vi "displayVolume.vi"(0 "frames":u16[][][](array[numeric]), 3 "z":dbl[](array[numeric]), 5 "overlay (z:-1 all planes)":cluster{"X":i32, "Y":i32, "Z":i32}[][](array[cluster]), 7 "stop immediately":bool) -> (13 "z profile":dbl[](array[numeric]), 14 "X0out":i32, 15 "deltaXout":i32, 16 "Y0out":i32, 17 "deltaYout":i32, 18 "zout (plane index)":i32 min=0 max=0)   [LabVIEW 2017]
uses:
  globalUtilities.vi
  <vilib>/Utility/file.llb/Write Delimited Spreadsheet (I64).vi
  <vilib>/Utility/file.llb/Write Delimited Spreadsheet (DBL).vi
  <vilib>/Analysis/NI_AALBase.lvlib
panel:
  in  "save marginal":bool
  in  "cut init frames":i32
  in  "refresh time (ms)":i32=200
  in  "zprof_variance":bool
  in  "save z profile":bool
  out "marginal plot":dbl[](graph)
  in  "marginal":u16(ring)=2 items=["x", "y", "none"]
  in  "z min":u16=100
  in  "z max":u16=65535
  in  "overlay depth":i32=3
  in  "overlay dotsize":i32=3
  in  "adjust y scale (to area)":bool
  out "Delta z":dbl
  in  "adjust y scale (to cursors)":bool
  out "single frame":T1(plugin-control)
  out "z profile of area":cluster{"X":dbl, "Y":dbl}[](graph)
  in  "deltaY":i32=4
  in  "deltaX":i32=8
  in  "Y0":i32=544
  in  "X0":i32=216
  out "single frame":u16[][](graph)
  in  "plane index":i32 min=0 max=37 format="%04.0f"
  out "axis-summed frame":u64[][](graph)
  in  "axis":u16(ring)=2 items=["x", "y", "z"]
  in  "stop":bool
  # "USE THIS VI TO DISPLAY A VOLUME"
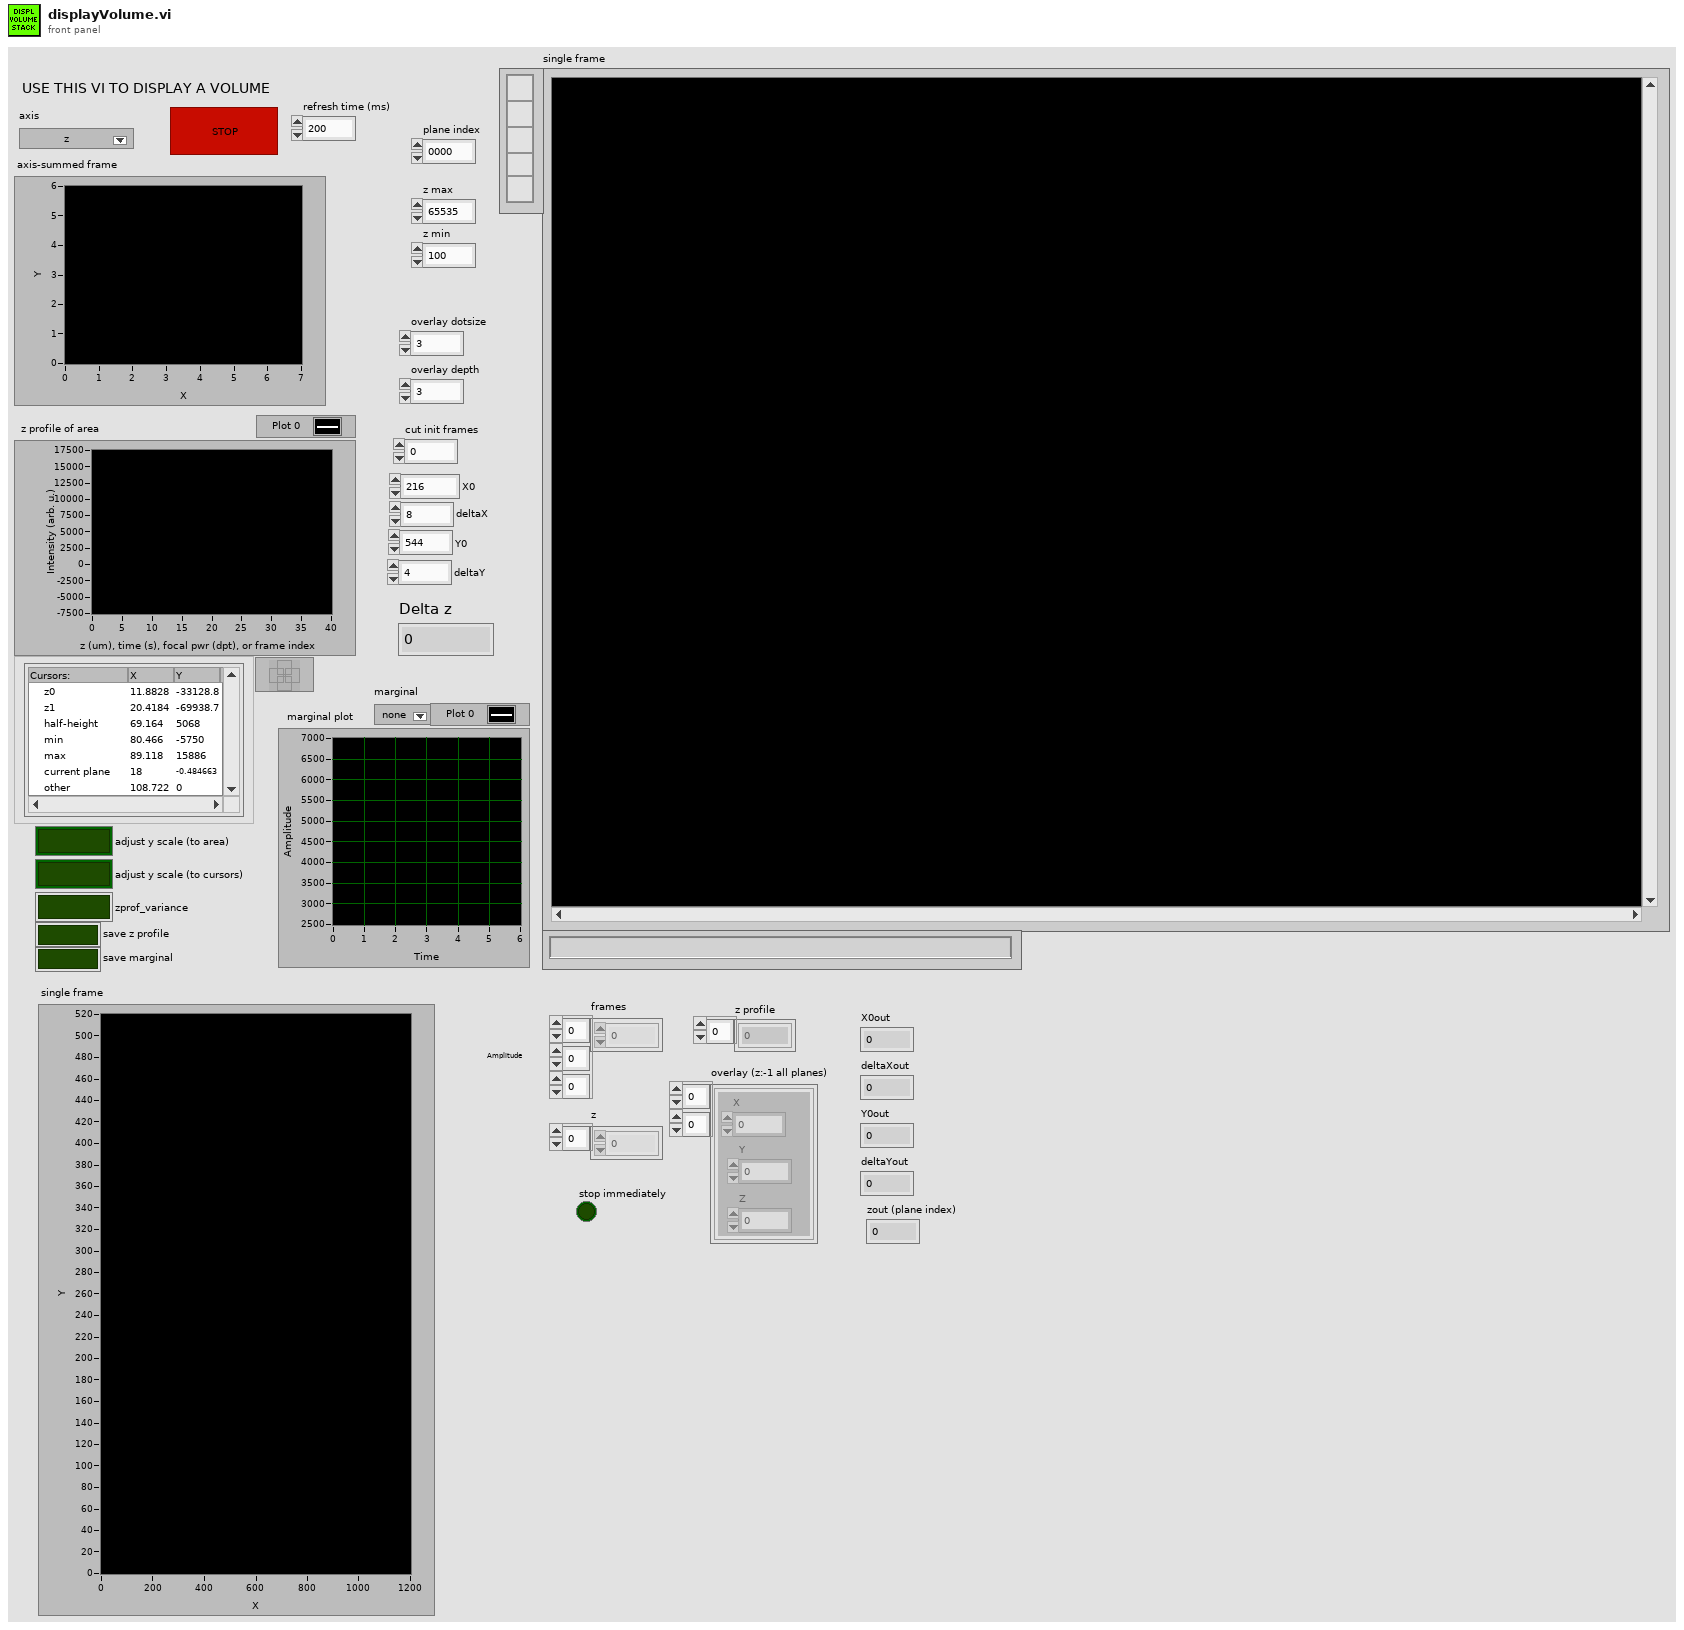
[diagram p1: front panel]
types:
  T1 = typedef "IMAQ Image.ctl" = refnum<image>
  T2 = typedef "Image Type" = u32
  T3 = typedef "LVCursorListTypeDef.ctl" = cluster{"Name":string, "Color":u32, "Style":u8, "Point Style":u8, "Name Visible":bool, "Allow Drag":bool, "Cursor Mode":u32, "Plot":i32, "Index":i32, "Position":cluster{"X":dbl, "Y":dbl}, "X Scale":u32, "Y Scale":u32, "Watch Plots":i32[], "Watch All Plots":bool, "Plot Area":i32, "Label Offset":cluster{"X":dbl, "Y":dbl}}[]
  T4 = cluster{"Name":string, "Color":u32, "Style":u8, "Point Style":u8, "Name Visible":bool, "Allow Drag":bool, "Cursor Mode":u32, "Plot":i32, "Index":i32, "Position":cluster{"X":dbl, "Y":dbl}, "X Scale":u32, "Y Scale":u32, "Watch Plots":i32[], "Watch All Plots":bool, "Plot Area":i32, "Label Offset":cluster{"X":dbl, "Y":dbl}}
  T5 = cluster{"Global Rectangle":i32[], "Contours":cluster{"Contour Type":u32, "ROI Type":u32, "Points":i32[]}[]}
  T6 = typedef "IMAQ Point" = cluster{"X":sgl, "Y":sgl}
  T7 = typedef "IMAQ Rectangle" = cluster{"Left":i32, "Top":i32, "Right":i32, "Bottom":i32, "Rotation":dbl}
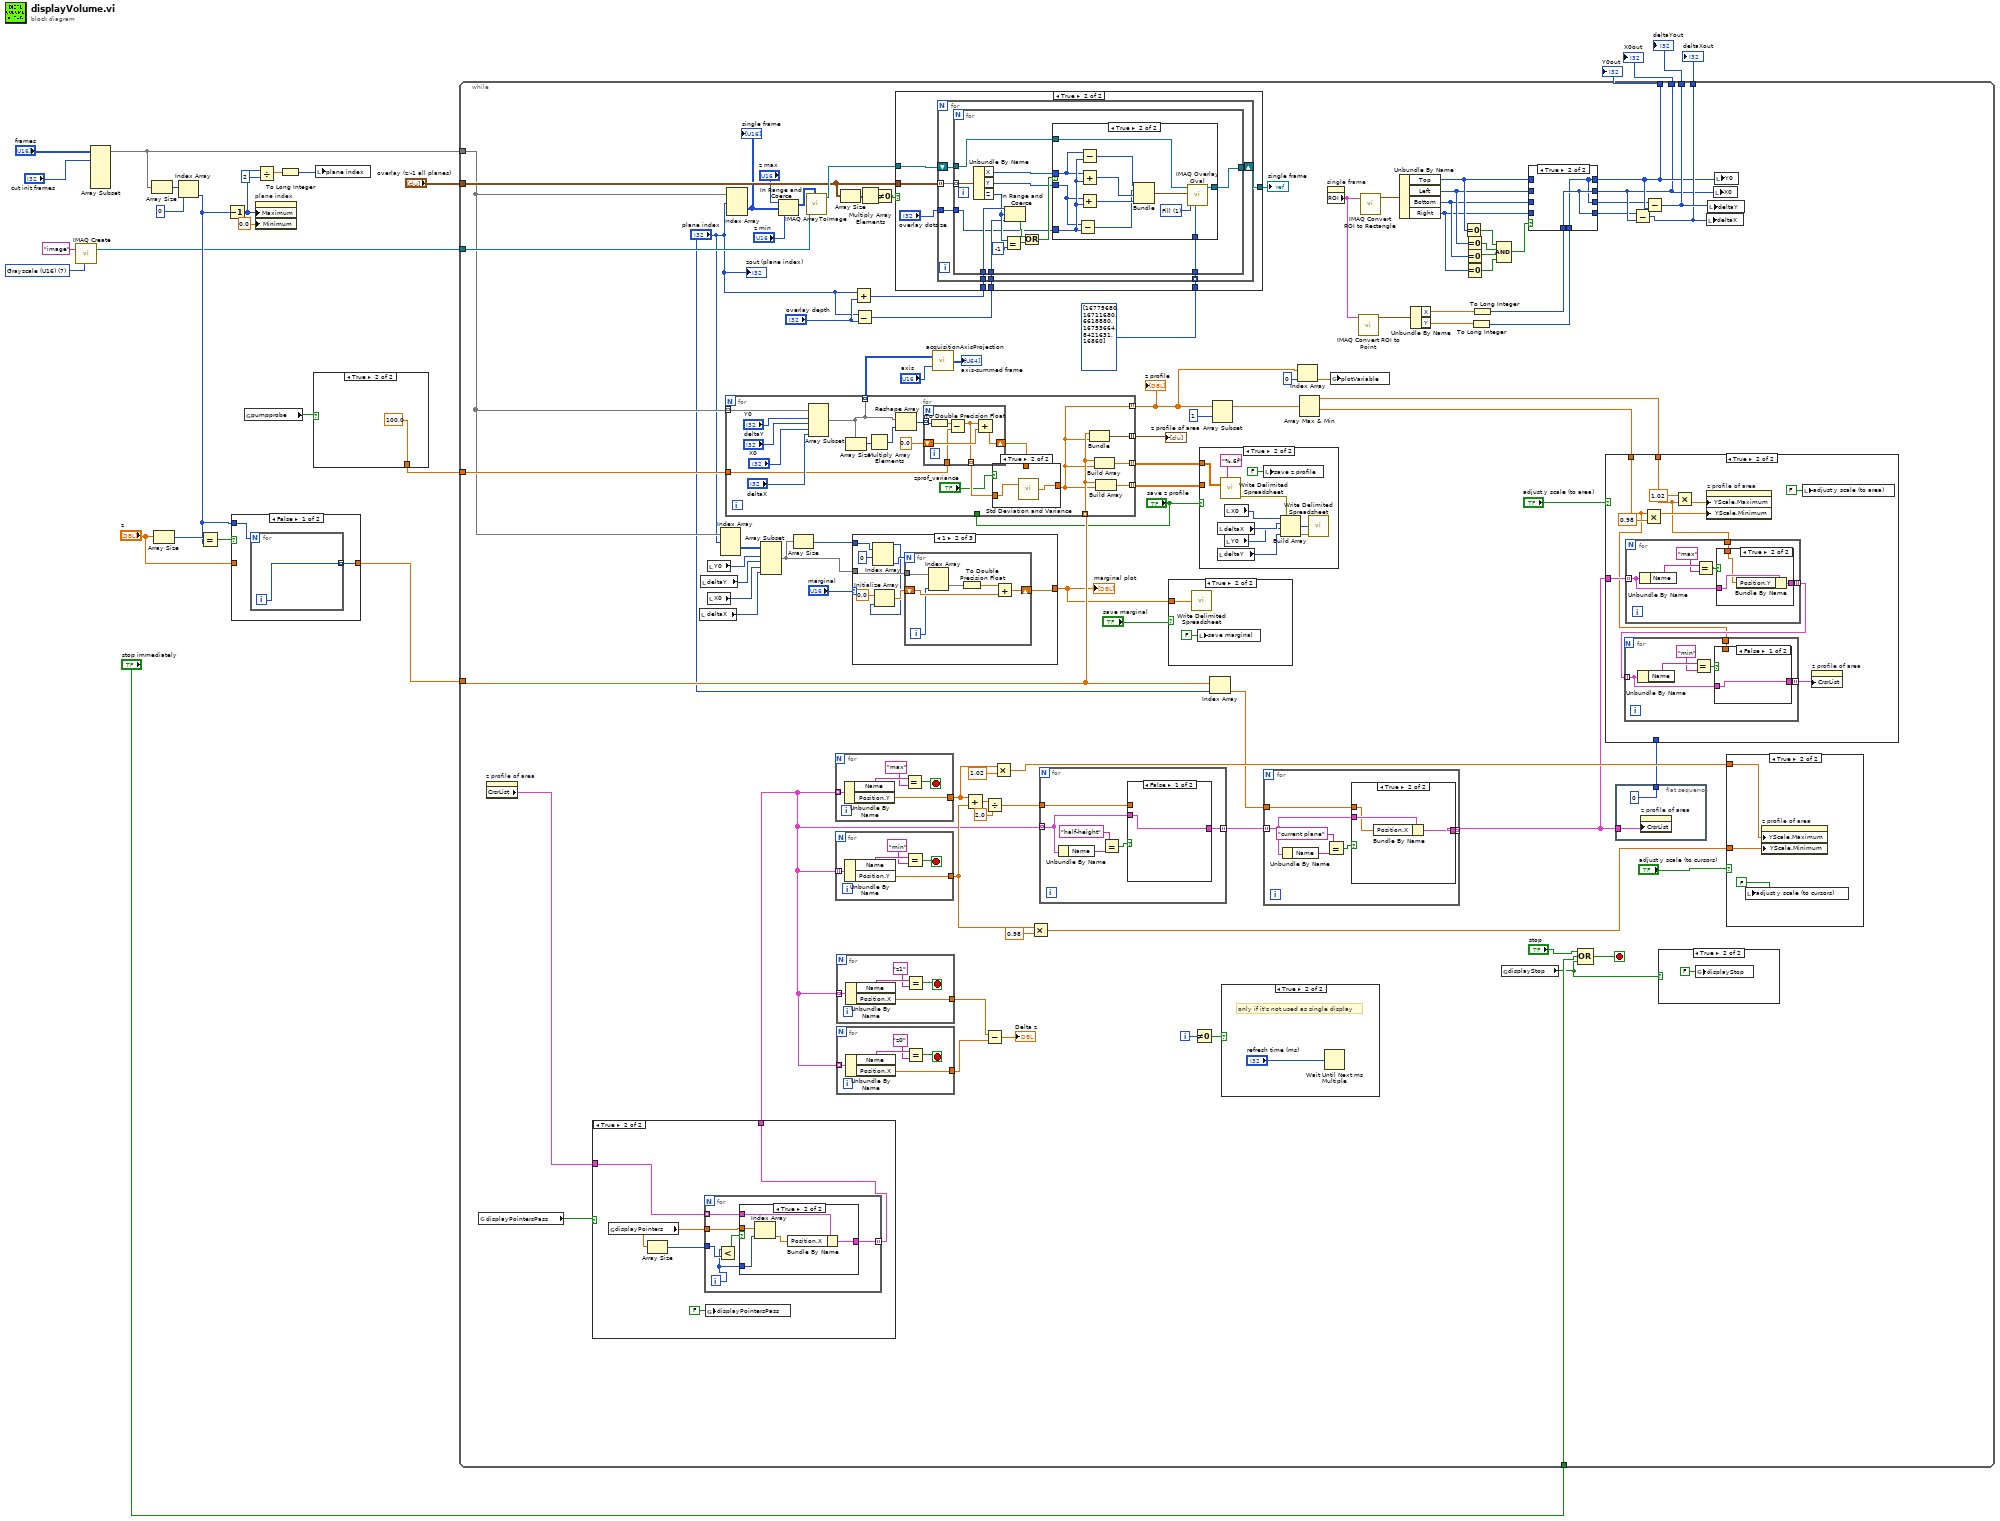
[diagram p0: block diagram]
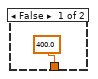
[diagram p2: hidden frame]
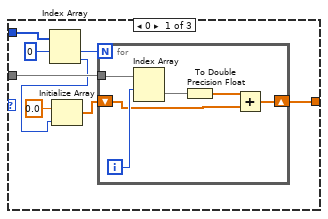
[diagram p10: hidden frame]
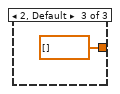
[diagram p11: hidden frame]
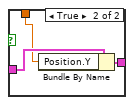
[diagram p17: hidden frame]
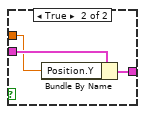
[diagram p20: hidden frame]
diagram:
  w19 = T2 7 items=["Grayscale (U8)", "Grayscale (I16)", "Grayscale (SGL)", "Complex (CSG)", "RGB (U32)", "HSL (U32)", "RGB (U64)", "Grayscale (U16)"] ("Image Type")
  n1 = call "IMAQ Create"("Image Name"="image", "Image Type"=w19) -> ("New Image"=w12:T1)  [unwired: 3 in, 1 out]
  n2 = Array Subset(array="frames", index (dim 0)="cut init frames") -> (w2:u16[][][])  [unwired: 5 in]
  n3 = Array Size(array=w2) -> (size(s)=w26:i32[])
  n4 = Array Size(array="z") -> (size(s)=w24:i32)
  n5 = Index Array(array=w26, index=0) -> (element=w18:i32)
  n6 = Equal?(x=w24, y=w18) -> (x = y?=w23:bool)
  n7 = Decrement(x=w18) -> (x-1=w6:i32)
  n8 = case shown="False" w23 {
    tunnel: [w27 w30] -> w21
    tunnel: "z" -> [_ w30]
    tunnel: w18 -> [w28 _]
    frame False {
      n9 = for {
        N: w28 -> [_]
        tunnel: [w29] -> w27 mode=indexing
        i -> [w29]
      }
    }
    frame True {
    }
  }
  n10 = global read "globalUtilities.vi" "pumpprobe"() -> (w8:bool)
  n11 = property on="plane index" class="DigNum (strict)"("Maximum"=w6, "Minimum"=0.0 ("Data Entry Limits:Minimum")) -> ()  [unwired: 2 in, 2 out]
  n12 = Divide(x=w6, y=2) -> (x/y=w10:dbl)
  n13 = To Long Integer(number=w10) -> (32bit integer=w9:i32)
  n14 = case shown="True" w8 {
    tunnel: [400.0 ("y") 100.0 ("y")] -> w7
    frame False {
    }
    frame True {
    }
  }
  n15 = local write "plane index"(w9) -> ()
  n16 = while {
    tunnel: w2 -> [w56]
    tunnel: w21 -> [w104]
    tunnel: w12 -> [w95]
    tunnel: [w84] -> w16
    tunnel: [w83] -> w15
    tunnel: [w97] -> w14
    tunnel: [w96] -> w13
    tunnel: "overlay (z:-1 all planes)" -> [w76]
    tunnel: w7 -> [w66]
    tunnel: "stop immediately" -> [w42]
    i -> [w39]
    stop <- w41 stop-if-true
    n17 = global read "globalUtilities.vi" "displayPointersPass"() -> (w37:bool)
    n18 = property on="z profile of area" class="XYGraph (strict)"() -> ("CrsrList"=w36:T3)  [unwired: 2 in, 2 out]
    n19 = case shown="True" w37 {
      tunnel: w36 -> [w127 w131]
      tunnel: [w127 w128] -> w35
      frame False {
      }
      frame True {
        n20 = global read "globalUtilities.vi" "displayPointers"() -> (w129:dbl[])
        n21 = Array Size(array=w129) -> (size(s)=w130:i32)
        n22 = for {
          tunnel: w131 -> [w138] mode=indexing
          tunnel: [w137] -> w128 mode=indexing
          tunnel: w130 -> [w136]
          tunnel: w129 -> [w134]
          i -> [w133]
          n23 = Less?(x=w133, y=w136) -> (x < y?=w135:bool)
          n24 = case shown="True" w135 {
            tunnel: w138 -> [w139 w144]
            tunnel: [w139 w143] -> w137
            tunnel: w134 -> [_ w142]
            tunnel: w133 -> [_ w141]
            frame False {
            }
            frame True {
              n25 = Index Array(array=w142, index=w141) -> (element=w140:dbl)
              n26 = Bundle By Name(cluster=w144, "Position.X"=w140) -> (w143:T4)
            }
          }
        }
        n27 = global write "globalUtilities.vi" "displayPointersPass"(FALSE ("displayPointersPass")) -> ()
      }
    }
    n28 = local read "deltaX"() -> (w50:i32)
    n29 = local read "deltaY"() -> (w52:i32)
    n30 = local read "Y0"() -> (w53:i32)
    n31 = local read "X0"() -> (w51:i32)
    n32 = Index Array(array=w56, index (dim 0)="plane index") -> (element=w54:u16[][])  [unwired: 2 in]
    n33 = for {
      tunnel: w56 -> [w326] mode=indexing
      tunnel: w104 -> [w312] mode=indexing
      tunnel: [w322] -> w122 mode=indexing
      tunnel: [w315] -> w70 mode=indexing
      tunnel: [w308] -> w58 mode=indexing
      tunnel: w66 -> [w317]
      tunnel: [w314] -> w47 mode=indexing
      tunnel: "save z profile" -> [_]
      tunnel: [w311] -> w45 mode=indexing
      n34 = Array Subset(array=w326, index (row)="Y0", length (row)="deltaY", index (col)="X0", length (col)="deltaX") -> (w315:u16[][])
      n35 = Array Size(array=w315) -> (size(s)=w316:i32[])
      n36 = Multiply Array Elements(1:w316) -> (0:w325:i32)
      n37 = Reshape Array(w315, w325) -> (w324:u16[])
      n38 = for {
        tunnel: w324 -> [w335] mode=indexing
        shift-right: [w333] -> w309
        shift-left: 0.0 -> [w334]
        tunnel: w317 -> [w331]
        tunnel: [w330] -> w313 mode=indexing
        n39 = To Double Precision Float(number=w335) -> (double precision float=w332:dbl)
        n40 = Subtract(x=w332, y=w331) -> (x-y=w330:dbl)
        n41 = Add(x=w330, y=w334) -> (x+y=w333:dbl)
      }
      n42 = case shown="True" "zprof_variance" {
        tunnel: w313 -> [_ w329]
        tunnel: [w327 w328] -> w308
        tunnel: w309 -> [w327 _]
        frame False {
        }
        frame True {
          n43 = call <vilib>:"Std Deviation and Variance.vi"("X"=w329) -> ("standard deviation"=w328:dbl)  [unwired: 1 in, 2 out]
        }
      }
      n44 = Bundle("Numeric"=w312, "standard deviation"=w308) -> (w322:cluster{"Numeric":dbl, "standard deviation":dbl})  [unwired: 1 in]
      n45 = Build Array(w312, w308) -> (w314:dbl[])
      n46 = Build Array(w312, w308) -> (w311:dbl[])
    }
    "z profile of area" <- w122
    "z profile" <- w58
    n47 = Index Array(array=w56, index (dim 0)="plane index") -> (element=w63:u16[][])  [unwired: 2 in]
    "single frame" <- w63
    n48 = Array Subset(array=w54, index (row)=w53, length (row)=w52, index (col)=w51, length (col)=w50) -> (w49:u16[][])
    n49 = In Range and Coerce(upper limit="z max", x=w63, lower limit="z min") -> (coerced(x)=w60:u16[][])  [unwired: 1 out]
    n50 = Array Size(array=w49) -> (size(s)=w48:i32[])
    n51 = call "IMAQ ArrayToImage"("Image Pixels (U16)"=w60, "Image"=w95) -> ("Image Out"=w93:T1)  [unwired: 8 in, 1 out]
    n52 = for {
      tunnel: w35 -> [w307] mode=indexing
      tunnel: [w303] -> w115
      stop <- w304 stop-if-true
      n53 = Unbundle By Name(w307) -> ("Name"=w306:string, "Position.Y"=w303:dbl)
      n54 = Equal?(x=w306, y="max") -> (x = y?=w304:bool)
    }
    n55 = for {
      tunnel: w35 -> [w302] mode=indexing
      tunnel: [w298] -> w117
      stop <- w299 stop-if-true
      n56 = Unbundle By Name(w302) -> ("Name"=w301:string, "Position.Y"=w298:dbl)
      n57 = Equal?(x=w301, y="min") -> (x = y?=w299:bool)
    }
    n58 = for {
      tunnel: w35 -> [w284] mode=indexing
      tunnel: [w280] -> w110
      stop <- w281 stop-if-true
      n59 = Unbundle By Name(w284) -> ("Name"=w283:string, "Position.X"=w280:dbl)
      n60 = Equal?(x=w283, y="z1") -> (x = y?=w281:bool)
    }
    n61 = for {
      tunnel: w35 -> [w279] mode=indexing
      tunnel: [w275] -> w109
      stop <- w276 stop-if-true
      n62 = Unbundle By Name(w279) -> ("Name"=w278:string, "Position.X"=w275:dbl)
      n63 = Equal?(x=w278, y="z0") -> (x = y?=w276:bool)
    }
    n64 = Array Size(array=w76) -> (size(s)=w75:i32[])
    n65 = case shown="1" "marginal" {
      tunnel: w48 -> [w165 w175 _]
      tunnel: w49 -> [w163 w176 _]
      tunnel: [w159 w177 dbl[] []] -> w33
      frame 0 {
        n66 = Index Array(array=w165, index #1=0 ("index")) -> (element #1=w161:i32, element #2=w158:i32)  [unwired: 1 in]
        n67 = Initialize Array(0.0 ("element"), w158) -> (w160:dbl[])
        n68 = for {
          N: w161 -> [_]
          tunnel: w163 -> [w171]
          shift-right: [w166] -> w159
          shift-left: w160 -> [w167]
          i -> [w170]
          n69 = Index Array(array=w171, index (row)=w170) -> (element=w169:u16[])  [unwired: 1 in]
          n70 = To Double Precision Float(number=w169) -> (double precision float=w168:dbl[])
          n71 = Add(x=w168, y=w167) -> (x+y=w166:dbl[])
        }
      }
      frame 1 {
        n72 = Index Array(array=w175, index #1=0 ("index")) -> (element #1=w172:i32, element #2=w173:i32)  [unwired: 1 in]
        n73 = Initialize Array(0.0 ("element"), w172) -> (w179:dbl[])
        n74 = for {
          N: w173 -> [_]
          tunnel: w176 -> [w185]
          shift-right: [w181] -> w177
          shift-left: w179 -> [w182]
          i -> [w180]
          n75 = Index Array(array=w185, index (col)=w180) -> (element=w184:u16[])  [unwired: 1 in]
          n76 = To Double Precision Float(number=w184) -> (double precision float=w183:dbl[])
          n77 = Add(x=w183, y=w182) -> (x+y=w181:dbl[])
        }
      }
      frame 2, Default {
      }
    }
    "marginal plot" <- w33
    n78 = Add(x="plane index", y="overlay depth") -> (x+y=w68:i32)
    n79 = Subtract(x="plane index", y="overlay depth") -> (x-y=w67:i32)
    n80 = Multiply Array Elements(1:w75) -> (0:w65:i32)
    n81 = Not Equal To 0?(x=w65) -> (x != 0?=w74:bool)
    n82 = case shown="True" w74 {
      tunnel: [w187 w193] -> w94
      tunnel: w93 -> [w187 w192]
      tunnel: w76 -> [_ w191]
      tunnel: w68 -> [_ w190]
      tunnel: w67 -> [_ w189]
      tunnel: u32[] [16775680, 16711680, 6618880, 16753664, 8421631, 16860] -> [_ w188]
      frame False {
      }
      frame True {
        n83 = for {
          tunnel: "overlay dotsize" -> [w201]
          tunnel: w191 -> [w198] mode=indexing
          tunnel: w190 -> [w197]
          tunnel: w189 -> [w196]
          shift-right: [w200] -> w193
          shift-left: w192 -> [w199]
          tunnel: w188 -> [w195] mode=indexing
          n84 = for {
            tunnel: w198 -> [w215] mode=indexing
            tunnel: w199 -> [w214]
            tunnel: w201 -> [w202]
            tunnel: [w213] -> w200
            tunnel: w197 -> [w212]
            tunnel: w196 -> [w209]
            tunnel: w195 -> [w203]
            n85 = Unbundle By Name(w215) -> ("X"=w205:i32, "Y"=w204:i32, "Z"=w211:i32)
            n86 = Equal?(x=w211, y=-1) -> (x = y?=w207:bool)
            n87 = In Range and Coerce(upper limit=w212, x=w211, lower limit=w209) -> (In Range?=w208:bool)  [unwired: 1 out]
            n88 = Or(x=w208, y=w207) -> (x .or. y?=w206:bool)
            n89 = case shown="True" w206 {
              tunnel: w214 -> [w216 w222]
              tunnel: w202 -> [_ w221]
              tunnel: [w216 w220] -> w213
              tunnel: w205 -> [_ w219]
              tunnel: w204 -> [_ w218]
              tunnel: w203 -> [_ w217]
              frame False {
              }
              frame True {
                w228 = u32 1 items=["Frame", "Fill"] ("Drawing Mode (Frame)")
                n90 = Subtract(x=w218, y=w221) -> (x-y=w224:i32)
                n91 = Add(x=w218, y=w221) -> (x+y=w226:i32)
                n92 = Subtract(x=w219, y=w221) -> (x-y=w223:i32)
                n93 = Add(x=w219, y=w221) -> (x+y=w225:i32)
                n94 = Bundle(w223, w224, w225, w226) -> (w227:cluster{i32, i32, i32, i32})  [unwired: 1 in]
                n95 = call "IMAQ Overlay Oval"("Color"=w217, "Drawing Mode (Frame)"=w228, "Bounding Rectangle"=w227, "Image"=w222) -> ("Image Out"=w220:T1)  [unwired: 6 in, 1 out]
              }
            }
          }
        }
      }
    }
    "single frame" <- w94
    n96 = call "acquisitionAxisProjection.vi"("axis (z)"="axis", "z stack"=w70) -> ("projected img"=→"axis-summed frame":u64[][])
    n97 = Add(x=w115, y=w117) -> (x+y=w120:dbl)
    n98 = Divide(x=w120, y=2.0) -> (x/y=w118:dbl)
    n99 = Subtract(x=w110, y=w109) -> (x-y=→"Delta z":dbl)
    n100 = Multiply(x=w115, y=1.02) -> (x*y=w112:dbl)
    n101 = Multiply(x=w117, y=0.98) -> (x*y=w111:dbl)
    n102 = for {
      tunnel: w35 -> [w289] mode=indexing
      tunnel: w118 -> [w290]
      tunnel: [w288] -> w102 mode=indexing
      n103 = Unbundle By Name(w289) -> ("Name"=w293:string)
      n104 = Equal?(x="half-height" ("y"), y=w293) -> (x = y?=w291:bool)
      n105 = case shown="False" w291 {
        tunnel: w290 -> [_ w296]
        tunnel: w289 -> [w294 w297]
        tunnel: [w294 w295] -> w288
        frame False {
        }
        frame True {
          n106 = Bundle By Name(cluster=w297, "Position.Y"=w296) -> (w295:T4)
        }
      }
    }
    n107 = case shown="True" "save marginal" {
      tunnel: w33 -> [_ w126]
      frame False {
      }
      frame True {
        n108 = call-poly <vilib>:"Write Delimited Spreadsheet.vi"("1D data"=w126) -> ()  [unwired: 13 in, 2 out]
        n109 = local write "save marginal"(FALSE ("save marginal")) -> ()
      }
    }
    n110 = Not Equal To 0?(x=w39) -> (x != 0?=w38:bool)
    n111 = case shown="True" "save z profile" {
      tunnel: w47 -> [_ w149]
      tunnel: w45 -> [_ _]
      frame False {
      }
      frame True {
        n112 = local read "deltaX"() -> (w153:i32)
        n113 = local read "deltaY"() -> (w151:i32)
        n114 = call-poly <vilib>:"Write Delimited Spreadsheet.vi"("format (%.3f)"="%.6f", "2D data"=w149) -> ("error out"=w155:errorcluster)  [unwired: 12 in, 1 out]
        n115 = local read "X0"() -> (w154:i32)
        n116 = local read "Y0"() -> (w152:i32)
        n117 = local write "save z profile"(FALSE ("save z profile")) -> ()
        n118 = Build Array(w154, w153, w152, w151) -> (w150:i32[])
        n119 = call-poly <vilib>:"Write Delimited Spreadsheet.vi"("1D data"=w150, "error in (no error)"=w155) -> ()  [unwired: 12 in, 2 out]
      }
    }
    n120 = Index Array(array=w104, index="plane index") -> (element=w103:dbl)
    n121 = Array Subset(array=w58, index=1) -> (w99:dbl[])  [unwired: 1 in]
    n122 = case shown="True" w38 {
      frame False {
      }
      frame True {
        # "only if it's not used as single display"
        n123 = Wait Until Next ms Multiple(millisecond multiple="refresh time (ms)") -> ()  [unwired: 1 out]
      }
    }
    n124 = for {
      tunnel: w102 -> [w236] mode=indexing
      tunnel: w103 -> [w237]
      tunnel: [w235] -> w101 mode=indexing
      n125 = Unbundle By Name(w236) -> ("Name"=w240:string)
      n126 = Equal?(x="current plane" ("y"), y=w240) -> (x = y?=w238:bool)
      n127 = case shown="True" w238 {
        tunnel: w237 -> [_ w243]
        tunnel: w236 -> [w241 w244]
        tunnel: [w241 w242] -> w235
        frame False {
        }
        frame True {
          n128 = Bundle By Name(cluster=w244, "Position.X"=w243) -> (w242:T4)
        }
      }
    }
    n129 = Index Array(array=w58, index=0) -> (element=w59:dbl)
    n130 = Array Max & Min(array=w99) -> (max value=w106:dbl, min value=w100:dbl)  [unwired: 2 out]
    n131 = property on="single frame" class="ImageControl"() -> ("ROI"=w79:T5)  [unwired: 2 in, 2 out]
    n132 = global write "globalUtilities.vi" "plotVariable"(w59) -> ()
    n133 = call "IMAQ Convert ROI to Point"("ROI Descriptor"=w79) -> ("Point"=w73:T6)  [unwired: 8 in, 1 out]
    n134 = call "IMAQ Convert ROI to Rectangle"("ROI Descriptor"=w79) -> ("Rectangle"=w121:T7)  [unwired: 8 in, 1 out]
    n135 = Unbundle By Name(w121) -> ("Top"=w88:i32, "Left"=w87:i32, "Bottom"=w86:i32, "Right"=w85:i32)
    n136 = Unbundle By Name(w73) -> ("X"=w72:sgl, "Y"=w71:sgl)
    n137 = Equal To 0?(x=w88) -> (x = 0?=w92:bool)
    n138 = Equal To 0?(x=w87) -> (x = 0?=w91:bool)
    n139 = Equal To 0?(x=w86) -> (x = 0?=w90:bool)
    n140 = Equal To 0?(x=w85) -> (x = 0?=w89:bool)
    n141 = To Long Integer(number=w71) -> (32bit integer=w77:i32)
    n142 = To Long Integer(number=w72) -> (32bit integer=w78:i32)
    n143 = Compound Arithmetic op=AND(w92, w91, w90, w89) -> (w80:bool)
    n144 = global read "globalUtilities.vi" "displayStop"() -> (w40:bool)
    n145 = case shown="True" w80 {
      tunnel: w88 -> [w232 _]
      tunnel: w87 -> [w231 _]
      tunnel: w86 -> [w230 _]
      tunnel: w85 -> [w229 _]
      tunnel: [w232 w233] -> w84
      tunnel: [w231 w234] -> w83
      tunnel: [w230 w233] -> w82
      tunnel: [w229 w234] -> w81
      tunnel: w78 -> [_ w234]
      tunnel: w77 -> [_ w233]
      frame False {
      }
      frame True {
      }
    }
    n146 = Compound Arithmetic op=OR("stop", w42, w40) -> (w41:bool)
    n147 = case shown="True" "adjust y scale (to area)" {
      tunnel: w106 -> [_ w249]
      tunnel: w100 -> [_ w247]
      tunnel: w101 -> [_ w250]
      tunnel: w44 -> [_ _]
      frame False {
      }
      frame True {
        n148 = for {
          tunnel: w250 -> [w266] mode=indexing
          tunnel: w249 -> [w267]
          tunnel: [w265] -> w248 mode=indexing
          n149 = Unbundle By Name(w266) -> ("Name"=w270:string)
          n150 = Equal?(x=w270, y="max") -> (x = y?=w268:bool)
          n151 = case shown="True" w268 {
            tunnel: w267 -> [_ w273]
            tunnel: w266 -> [w271 w274]
            tunnel: [w271 w272] -> w265
            frame False {
            }
            frame True {
              n152 = Bundle By Name(cluster=w274, "Position.Y"=w273) -> (w272:T4)
            }
          }
        }
        n153 = for {
          tunnel: w248 -> [w256] mode=indexing
          tunnel: w247 -> [w257]
          tunnel: [w255] -> w246 mode=indexing
          n154 = Unbundle By Name(w256) -> ("Name"=w260:string)
          n155 = Equal?(x=w260, y="min") -> (x = y?=w258:bool)
          n156 = case shown="False" w258 {
            tunnel: w257 -> [_ w263]
            tunnel: w256 -> [w261 w264]
            tunnel: [w261 w262] -> w255
            frame False {
            }
            frame True {
              n157 = Bundle By Name(cluster=w264, "Position.Y"=w263) -> (w262:T4)
            }
          }
        }
        n158 = Multiply(x=w247, y=0.98) -> (x*y=w254:dbl)
        n159 = Multiply(x=1.02, y=w249) -> (x*y=w252:dbl)
        n160 = property on="z profile of area" class="XYGraph (strict)"("YScale.Maximum"=w252, "YScale.Minimum"=w254) -> ()  [unwired: 2 in, 2 out]
        n161 = local write "adjust y scale (to area)"(FALSE ("adjust y scale (to area)")) -> ()
        n162 = property on="z profile of area" class="XYGraph (strict)"("CrsrList"=w246) -> ()  [unwired: 2 in, 2 out]
      }
    }
    n163 = flat-sequence {
      tunnel: w101 -> [w148]
      tunnel: [0] -> w44
      frame #0 {
        n164 = property on="z profile of area" class="XYGraph (strict)"("CrsrList"=w148) -> ()  [unwired: 2 in, 2 out]
      }
    }
    n165 = Subtract(x=w81, y=w83) -> (x-y=w96:i32)
    n166 = Subtract(x=w82, y=w84) -> (x-y=w97:i32)
    n167 = case shown="True" w40 {
      frame False {
      }
      frame True {
        n168 = global write "globalUtilities.vi" "displayStop"(FALSE ("displayStop")) -> ()
      }
    }
    n169 = local write "deltaX"(w96) -> ()
    n170 = local write "deltaY"(w97) -> ()
    n171 = local write "X0"(w83) -> ()
    n172 = local write "Y0"(w84) -> ()
    n173 = case shown="True" "adjust y scale (to cursors)" {
      tunnel: w112 -> [_ w287]
      tunnel: w111 -> [_ w286]
      frame False {
      }
      frame True {
        n174 = local write "adjust y scale (to cursors)"(FALSE ("adjust z scale")) -> ()
        n175 = property on="z profile of area" class="XYGraph (strict)"("YScale.Maximum"=w287, "YScale.Minimum"=w286) -> ()  [unwired: 2 in, 2 out]
      }
    }
    "zout (plane index)" <- "plane index"
  }
  "Y0out" <- w16
  "X0out" <- w15
  "deltaYout" <- w14
  "deltaXout" <- w13
